vi "VG-close.vi"(11 "VG-VNA_GUI in":refnum<class "VG-VNA_GUI.lvclass">) -> (3 "VG-VNA_GUI out":refnum<class "VG-VNA_GUI.lvclass">)   [LabVIEW 2020, in "VG-VNA_GUI.lvlib" / "VG-VNA_GUI.lvclass"]
uses:
  VG-VNA_GUI.lvclass
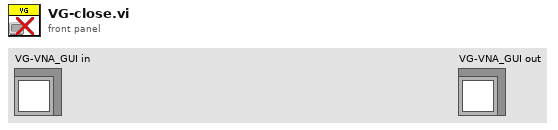
[diagram p1: front panel]
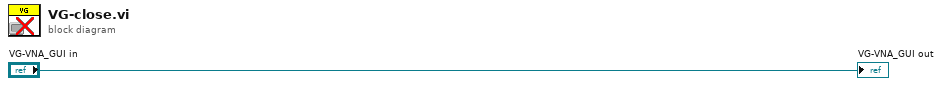
[diagram p0: block diagram]
diagram:
  "VG-VNA_GUI out" <- "VG-VNA_GUI in"
